vi "CreatSaveFile.vi"(8 "error in (no error)":errorcluster, 11 "Data_In":T1) -> (0 "error out":errorcluster, 2 "FileSave path":path, 3 "DataTable":string[][](array[string]), 5 "Data_out":T1)   [LabVIEW 2014]
uses:
  controls/Data1.ctl
  controls/Payjson.ctl
  <vilib>/Utility/file.llb/Write To Spreadsheet File (string).vi
  <vilib>/Utility/file.llb/Read From Spreadsheet File (string).vi
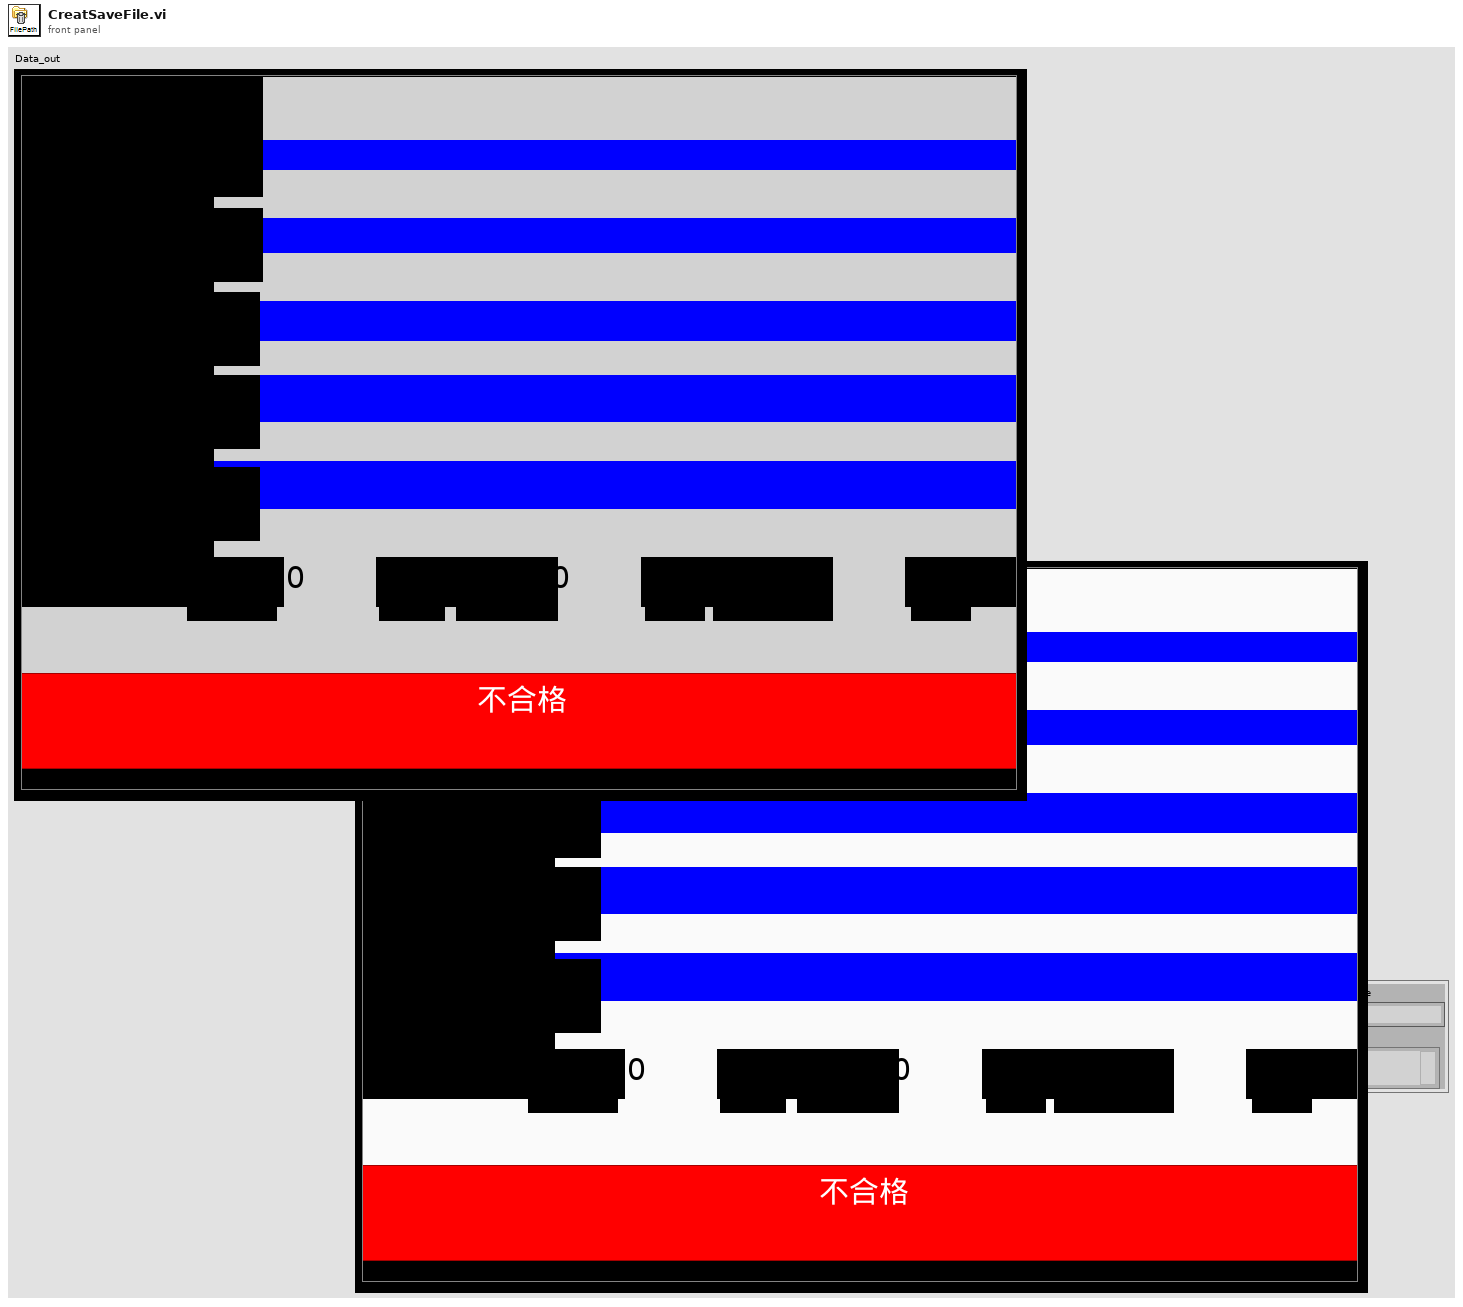
[diagram p1: front panel]
types:
  T1 = typedef "Data1.ctl" = cluster{"Date":string, "BarCode1":string, "BarCode2":string, "BarCode3":string, "Message":string, "OK Count":u16, "NG Count":u16, "Total Count":u16, "ModelData":string[][], "OK&NG":bool, "COM1":refnum<visa-resource-name>, "COM2":refnum<visa-resource-name>, "IO":i32, "Time":u32, "TCP":refnum<k5>, "TCP 2":refnum<k5>, "COM1 2":refnum<visa-resource-name>, "CheckNum":string, "BarCode1_1":string, "BarCode2_1":string, "BarCode3_1":string, "日期":string, "機種":string, "機號":string, "商品條碼1":string, "OK_1":string, "OK":string, "NG":string, "NG_1":string, "Total":string, "Total_1":string, "ClaerTime":u32, "Pjson":T2, "LotNo":string[], "CheckParsArray":string[], "BarCode4":string, "BarCode4_1":string, "商品條碼2":string, "BarCode5":string, "BarCode5_1":string, "商品條碼3":string, "ReScanNG":i32, "NGTimeCT":u32}
  T2 = typedef "Payjson.ctl" = cluster{"DEPT":string, "LINE":string, "STANO":string, "WORKNO":string, "PRODSN":string, "COMPNTID":string, "COMPNTLOT":string, "COMPNTSN":string, "USEDQTY":i16, "OPDATE":string, "OPUSER":string, "RECVDATE":string, "MMODU":string}[]
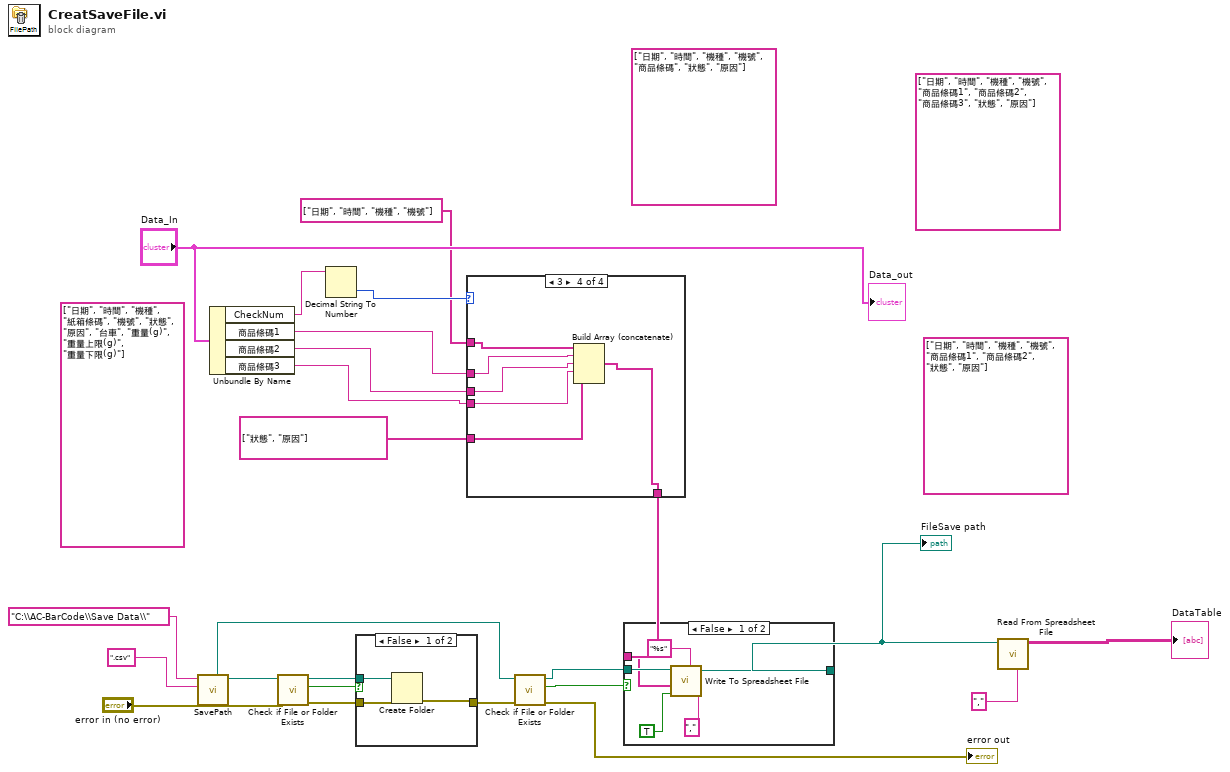
[diagram p0: block diagram]
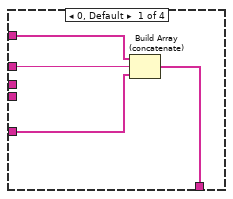
[diagram p2: hidden frame]
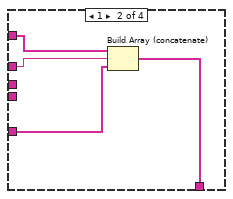
[diagram p3: hidden frame]
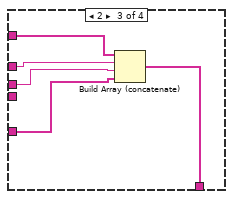
[diagram p4: hidden frame]
diagram:
  (unwired) string[] ["日期", "時間", "機種", "機號", "商品條碼1", "商品條碼2", "商品條碼3", "狀態", "原因"]
  (unwired) string[] ["日期", "時間", "機種", "機號", "商品條碼1", "商品條碼2", "狀態", "原因"]
  (unwired) string[] ["日期", "時間", "機種", "機號", "商品條碼", "狀態", "原因"]
  (unwired) string[] ["日期", "時間", "機種", "紙箱條碼", "機號", "狀態", "原因", "台車", "重量(g)", "重量上限(g)", "重量下限(g)"]
  n1 = call "SavePath.vi"("File Name"=".csv", "Path In"="C:\\AC-BarCode\\Save Data\\") -> ("Folder Path"=w24:path, "File Path"=w22:path)  [unwired: 8 in]
  n2 = Unbundle By Name("Data_In") -> ("CheckNum"=w9:string, "商品條碼1"=w4:string, "商品條碼2"=w2:string, "商品條碼3"=w1:string)
  n3 = call <vilib>:"Check if File or Folder Exists.vi"("error in (no error)"="error in (no error)", "path"=w24) -> ("error out"=w21:errorcluster, "file or folder exists?"=w23:bool, "dup path"=w19:path)  [unwired: 7 in]
  n4 = Decimal String To Number(string=w9) -> (number=w8:i32)  [unwired: 2 in, 1 out]
  n5 = case shown="False" w23 {
    tunnel: w21 -> [w26 w28]
    tunnel: [w25 w28] -> w20
    tunnel: w19 -> [w27 _]
    frame False {
      n6 = Create Folder(path (use dialog)=w27, error in=w26) -> (error out=w25:errorcluster)  [unwired: 1 in, 2 out]
    }
    frame True {
    }
  }
  n7 = case shown="3" w8 {
    tunnel: [w29 w33 w37 w42] -> w7
    tunnel: string[] ["日期", "時間", "機種", "機號"] -> [w32 w36 w41 w47]
    tunnel: w4 -> [w31 w35 w40 w46]
    tunnel: string[] ["狀態", "原因"] -> [w30 w34 w38 w43]
    tunnel: w2 -> [_ _ w39 w45]
    tunnel: w1 -> [_ _ _ w44]
    frame 0, Default {
      n8 = Build Array (concatenate)(w32, w31, w30) -> (w29:string[])
    }
    frame 1 {
      n9 = Build Array (concatenate)(w36, w35, w34) -> (w33:string[])
    }
    frame 2 {
      n10 = Build Array (concatenate)(w41, w40, w39, w38) -> (w37:string[])
    }
    frame 3 {
      n11 = Build Array (concatenate)(w47, w46, w45, w44, w43) -> (w42:string[])
    }
  }
  n12 = call <vilib>:"Check if File or Folder Exists.vi"("error in (no error)"=w20, "path"=w22) -> ("error out"=→"error out":errorcluster, "file or folder exists?"=w17:bool, "dup path"=w18:path)  [unwired: 7 in]
  n13 = case shown="False" w17 {
    tunnel: w18 -> [w53 w54]
    tunnel: [w51 w54] -> w10
    tunnel: w7 -> [w48 _]
    frame False {
      n14 = call-poly <vilib>:"Write To Spreadsheet File.vi"("delimiter (\\t)"="," ("delimiter (\\t)"), "format (%s)"="%s" ("format (%.3f)"), "append to file? (new file:F)"=TRUE, "1D data"=w48, "file path (dialog if empty)"=w53) -> ("new file path (Not A Path if cancelled)"=w51:path)  [unwired: 3 in]
    }
    frame True {
    }
  }
  "FileSave path" <- w10
  n15 = call-poly <vilib>:"Read From Spreadsheet File.vi"("delimiter (\\t)"="," ("delimiter (\\t)"), "file path (dialog if empty)"=w10) -> ("all rows"=→"DataTable":string[][])  [unwired: 5 in, 4 out]
  "Data_out" <- "Data_In"
